vi "EMS Black Start Status.vi"(4 "error":string, 6 "Status":T1, 8 "error in (no error)":errorcluster, 10 "Sequence":string, 11 "Master Controller in":refnum<class "Master Controller.lvclass">) -> (0 "error out":errorcluster, 3 "Master Controller out":refnum<class "Master Controller.lvclass">)   [LabVIEW 2015, in "Master Controller Core.lvlib" / "Master Controller.lvclass"]
uses:
  Master Controller.lvclass
  SCADA Core/SCADA Abstract Messages/Black Start Status Msg/Black Start Status.ctl
  Communications/SCADA Communcations Actor/SCADA Communications/Controls/EMS Message Cluster.ctl
  Master Controller.lvclass/Master Controller.ctl
  Communications/SCADA Communcations Actor/SCADA Communications Messages/Transmit EMS Message Msg/Transmit EMS Message Msg.lvclass/Transmit EMS Message Msg.ctl
  <vilib>/ActorFramework/Message Enqueuer/Message Enqueuer.lvclass/Message Enqueuer.ctl
  <vilib>/ActorFramework/Message Enqueuer/Enqueue.vi
  <vilib>/ActorFramework/Message Priority Queue/Priority Enqueue.vi
  Communications/SCADA Communcations Actor/SCADA Communications Messages/Transmit EMS Message Msg/Transmit EMS Message Msg.lvclass
  Communications/SCADA Communcations Actor/SCADA Communications/SCADA Communications.lvclass
  Utilities/Message Strings.llb/Message String Utilities.lvlib
  Utilities/Status Messaging.llb/Status Messaging.lvlib
  SCADA Core/SCADA Abstract Messages/Black Start Status Msg/Black Start Status Msg.lvclass
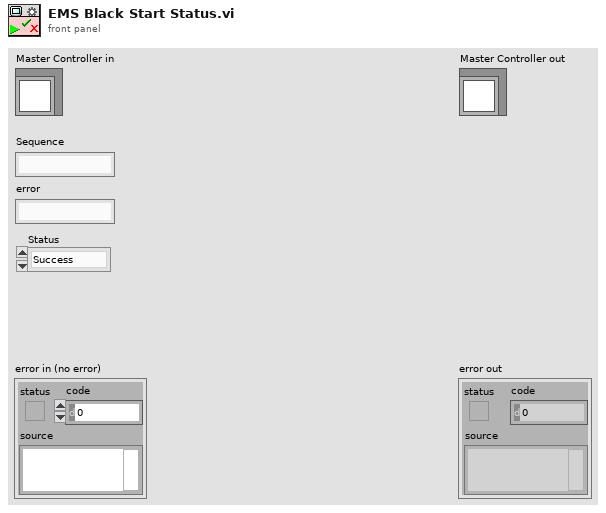
[diagram p1: front panel]
types:
  T1 = typedef "SCADA Core.lvlib/Black Start Status Msg.lvclass/Black Start Status.ctl" = enum16{"Success", "Failure"}
  T2 = typedef "SCADA Communcations Actor.lvlib/SCADA Communications.lvclass/EMS Message Cluster.ctl" = cluster{"Name":string, "Content":string}
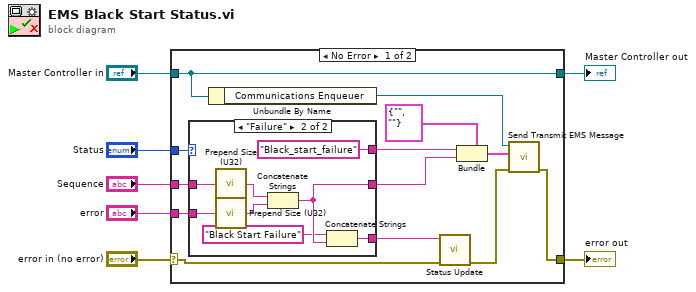
[diagram p0: block diagram]
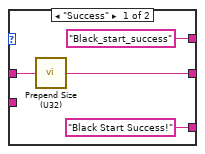
[diagram p2: hidden frame]
diagram:
  n1 = case shown="No Error" "error in (no error)" {
    selector: "error in (no error)" -> [w10 w34]
    tunnel: [w15 w34] -> w6
    tunnel: [w19 w33] -> w4
    tunnel: "Master Controller in" -> [w19 w33]
    tunnel: "error" -> [w13 _]
    tunnel: "Status" -> [w20 _]
    tunnel: "Sequence" -> [w12 _]
    frame No Error {
      n2 = case shown="\"Failure\"" w20 {
        tunnel: ["Black_start_success" ("Name") "Black_start_failure" ("Name")] -> w14
        tunnel: w13 -> [_ w31]
        tunnel: w12 -> [w23 w30]
        tunnel: [w22 w26] -> w11
        tunnel: ["Black Start Success!" ("Name") w27] -> w8
        frame "Success" {
          n3 = call "Prepend Size (U32).vi"("String in"=w23) -> ("String out"=w22:string)
        }
        frame "Failure" {
          n4 = call "Prepend Size (U32).vi"("String in"=w30) -> ("String out"=w28:string)
          n5 = call "Prepend Size (U32).vi"("String in"=w31) -> ("String out"=w29:string)
          n6 = Concatenate Strings(w28, w29) -> (w26:string)
          n7 = Concatenate Strings("Black Start Failure" ("Name"), w26) -> (w27:string)
        }
      }
      n8 = Unbundle By Name(w19) -> ("Communications Enqueuer"=w17:refnum<class "Message Enqueuer.lvclass">)
      n9 = call "Status Update.vi"("error in (no error)"=w10, "Status Update"=w8) -> ("error out"=w9:errorcluster)  [unwired: 8 in, 1 out]
      n10 = Bundle(cluster=T2 {"Name"="", "Content"=""} ("Message"), "Name"=w14, "Content"=w11) -> (w16:T2)
      n11 = call "Send Transmit EMS Message.vi"("error in (no error)"=w9, "Message"=w16, "Message Enqueuer"=w17) -> ("error out"=w15:errorcluster)  [unwired: 7 in, 1 out]
    }
    frame Error {
    }
  }
  "error out" <- w6
  "Master Controller out" <- w4
